vi "Config Bias.vi"(8 "error in":errorcluster, 10 "Bias (Off)":i32(ring) items=["Disabled", "100 megohm", "1 megohm"], 11 "VISA resource name":refnum<visa-resource-name>) -> (0 "error out":errorcluster, 3 "VISA resource name out":refnum<visa-resource-name>)   [LabVIEW 2018, in "Andeen-Hagerling 2700.lvlib"]
doc: "This VI enables or disables a user-supplied DC bias voltage of up to ±100 VDC to be applied to the measured unknown. The external source is connected to the rear panel DC BIAS input. This command also selects the value of an internal resistor that is placed in series with the externally applied voltage source."
uses:
  Andeen-Hagerling 2700.lvlib
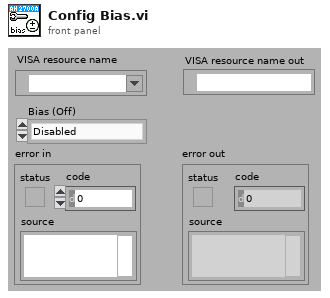
[diagram p1: front panel]
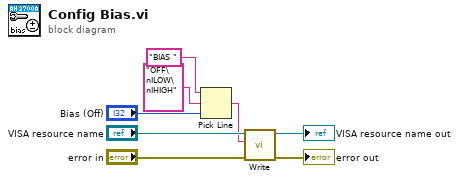
[diagram p0: block diagram]
diagram:
  n1 = Pick Line(string ("")="BIAS ", multi-line string="OFF\nILOW\nIHIGH", line index="Bias (Off)") -> (output string=w3:string)
  n2 = call "Write.vi"("error in"="error in", "command"=w3, "VISA resource name"="VISA resource name") -> ("error out"=→"error out":errorcluster, "VISA resource name out"=→"VISA resource name out":refnum<visa-resource-name>)  [unwired: 7 in]
